vi "Integrate to Velocity.vi"(1 "x":dbl) -> (0 "Output":dbl)   [LabVIEW 2017]
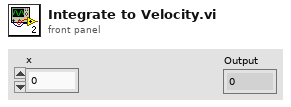
[diagram p1: front panel]
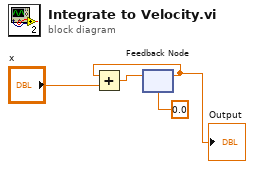
[diagram p0: block diagram]
diagram:
  n1 = feedback #1(0.0 ("x")) -> (w1:dbl)
  "Output" <- w1
  n2 = Add(x=w1, y="x") -> (x+y=w2:dbl)
  n3 = feedback-in #1(w2) -> ()
